vi "pong for x (SubVI).vi"(6 "Pilka uderzyla w paletke":bool, 7 "Numeric in":i32, 8 "loakcja x":i32, 11 "szybkosc x":i32) -> (0 "lokacja x wyjsciowa":i32, 1 "Pilka uderzyla w lewa sciane":bool, 2 "Pilka uderzyla w prawa sciane":bool, 3 "szybkosc x wyjsciowa":i32, 5 "Pilka uderzyla w prawa lub lewa sicane":bool)   [LabVIEW 2018]
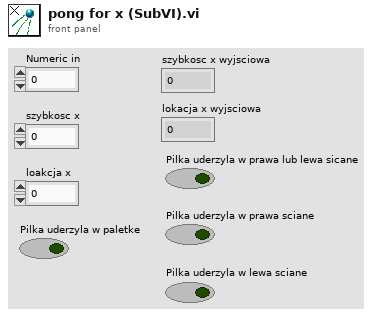
[diagram p1: front panel]
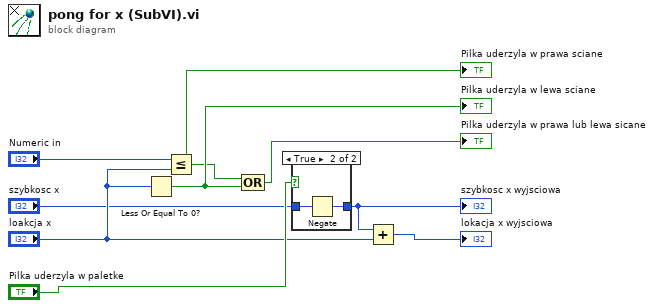
[diagram p0: block diagram]
diagram:
  n1 = Less Or Equal To 0?(x="loakcja x") -> (x <= 0?=w8:bool)
  "Pilka uderzyla w lewa sciane" <- w8
  n2 = Less Or Equal?(x="Numeric in", y="loakcja x") -> (x <= y?=w7:bool)
  "Pilka uderzyla w prawa sciane" <- w7
  n3 = Compound Arithmetic op=OR(w7, w8) -> (→"Pilka uderzyla w prawa lub lewa sicane":bool)
  n4 = case shown="True" "Pilka uderzyla w paletke" {
    tunnel: "szybkosc x" -> [w10 w12]
    tunnel: [w10 w11] -> w6
    frame False {
    }
    frame True {
      n5 = Negate(x=w12) -> (-x=w11:i32)
    }
  }
  "szybkosc x wyjsciowa" <- w6
  n6 = Add(x=w6, y="loakcja x") -> (x+y=→"lokacja x wyjsciowa":i32)
